vi "Alarm Type Encode.vi"(1 "Input":dbl min=-10000.0 max=10000.0 step=0.001) -> (0 "resulting string":string)   [LabVIEW 2024]
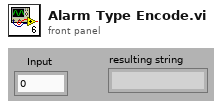
[diagram p1: front panel]
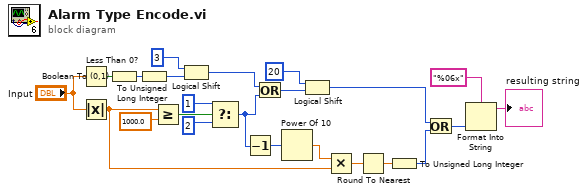
[diagram p0: block diagram]
diagram:
  n1 = Less Than 0?(x="Input") -> (x < 0?=w22:bool)
  n2 = Absolute Value(x="Input") -> (abs(x)=w8:dbl)
  n3 = Boolean To (0,1)(Boolean=w22) -> (0, 1=w21:i16)
  n4 = To Unsigned Long Integer(number=w21) -> (unsigned 32bit integer=w20:u32)
  n5 = Greater Or Equal?(x=w8, y=1000.0) -> (x >= y?=w17:bool)
  n6 = Logical Shift(y=u32 3, x=w20) -> (x << y=w14:u32)
  n7 = Select(t=u32 1, s=w17, f=u32 2) -> (s? t:f=w11:u32)
  n8 = Decrement(x=w11) -> (x-1=w10:u32)
  n9 = Or(x=w14, y=w11) -> (x .or. y?=w12:u32)
  n10 = Power Of 10(x=w10) -> (10^x=w9:dbl)
  n11 = Logical Shift(y=u32 20, x=w12) -> (x << y=w6:u32)
  n12 = Multiply(x=w9, y=w8) -> (x*y=w7:dbl)
  n13 = Round To Nearest(number=w7) -> (nearest integer value=w5:dbl)
  n14 = To Unsigned Long Integer(number=w5) -> (unsigned 32bit integer=w4:u32)
  n15 = Or(x=w6, y=w4) -> (x .or. y?=w3:u32)
  n16 = Format Into String(format string="%06x", w3) -> (resulting string=→"resulting string":string)  [unwired: 2 in, 1 out]
